vi "Read-all-variables.vi"(8 "error in (no error)":errorcluster, 11 "Acquis. params. ref. in":refnum<data-value>) -> (0 "error out":errorcluster, 2 "Acquis. vars.":T1, 3 "Acquis. params. ref.":refnum<data-value>)   [LabVIEW 2013, in "CameraVision.lvlib" / "CV-Acquisition.lvclass"]
uses:
  CV-Acquisition.lvclass
  Acquisition-variables.ctl
  UI/Module-states.ctl
  CV-Acquisition.lvclass/CV-Acquisition.ctl
  UI/CV-UI.lvclass
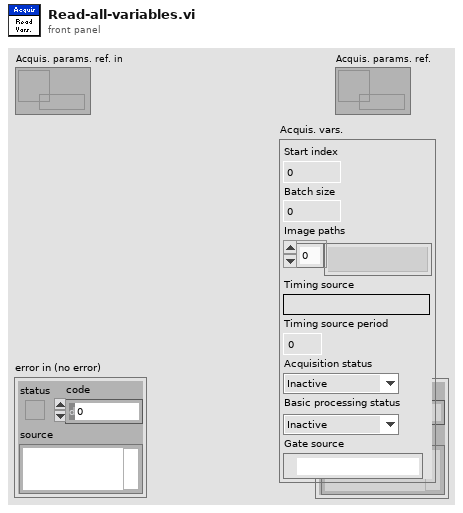
[diagram p1: front panel]
types:
  T1 = typedef "CameraVision.lvlib/CV-Acquisition.lvclass/Acquisition-variables.ctl" = cluster{"Start index":i32, "Batch size":i32, "Image paths":path[], "Timing source":string, "Timing source period":i64, "Acquisition status":T2, "Basic processing status":T2, "Gate source":refnum<k21>}
  T2 = typedef "CameraVision.lvlib/CV-UI.lvclass/Module-states.ctl" = enum16{"Inactive", "Active", "Data-loss", "Error", "Simulation", "Synchronizing", "Initialized", "Released"}
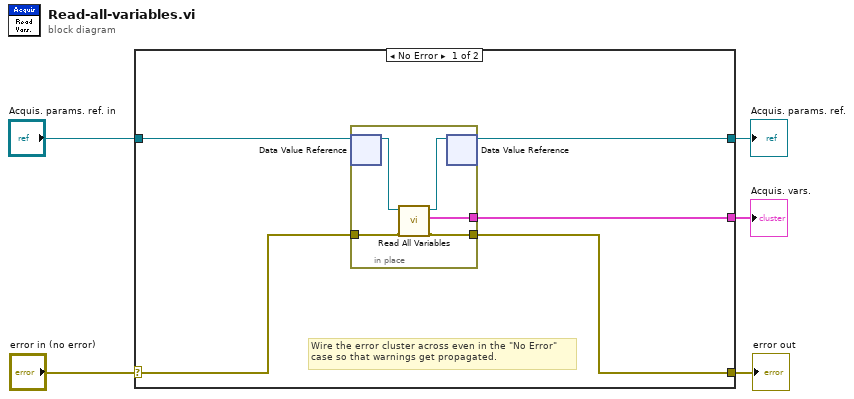
[diagram p0: block diagram]
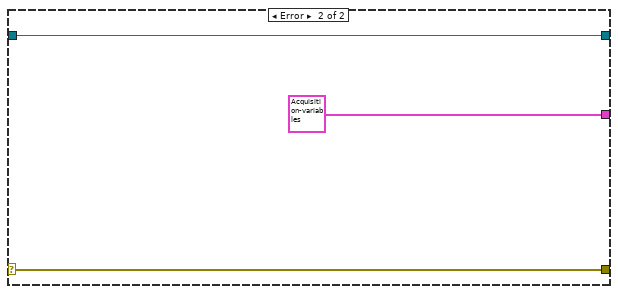
[diagram p2: hidden frame]
diagram:
  n1 = case shown="No Error" "error in (no error)" {
    selector: "error in (no error)" -> [w10 w18]
    tunnel: [w9 w18] -> w4
    tunnel: "Acquis. params. ref. in" -> [w7 w16]
    tunnel: [w8 T1 {"Start index"=0, "Batch size"=0, "Image paths"=[], "Timing source"="", "Timing source period"=0, "Acquisition status"=enum."Inactive", "Basic processing status"=enum."Inactive", "Gate source"=""} ("Acquis. vars.")] -> w2
    tunnel: [w6 w16] -> w1
    frame No Error {
      # "Wire the error cluster across even in the \"No Error\"\ncase so that warnings get propagated."
      n2 = in-place {
        in-place-border: w10 -> [w15]
        in-place-border: [w14] -> w9
        in-place-border: [w13] -> w8
        n3 = in-place-dvr #1(w7) -> (w12:refnum<class "CV-Acquisition.lvclass">)  [unwired: 1 out]
        n4 = call "Read All Variables.vi"("error in (no error)"=w15, "Acquis params in"=w12) -> ("error out"=w14:errorcluster, "Acquis. vars."=w13:T1, "Acquis params out"=w11:refnum<class "CV-Acquisition.lvclass">)  [unwired: 7 in]
        n5 = in-place-dvr #1(w11) -> (w6:refnum<data-value>)  [unwired: 1 out]
      }
    }
    frame Error {
    }
  }
  "error out" <- w4
  "Acquis. params. ref." <- w1
  "Acquis. vars." <- w2
